vi "test hidde panel.vi"(8 "error in (no error)":errorcluster, 11 "TestCase in":refnum<class "Test Osciloscope Module.lvclass">) -> (0 "error out":errorcluster, 3 "TestCase out":refnum<class "Test Osciloscope Module.lvclass">)   [LabVIEW 2020, in "Test Osciloscope Module.lvclass"]
uses:
  Test Osciloscope Module.lvclass
  Test Osciloscope Module.lvclass/Test Osciloscope Module.ctl
  <vilib>/addons/_JKI Toolkits/VI Tester/TestCase.llb/TestCase.lvclass
  Libraries/Osciloscope/Osciloscope.lvlib
  C:/Program Files (x86)/National Instruments/LabVIEW 2020/vi.lib/addons/_JKI Toolkits/VI Tester/TestCase.llb/TestCase.lvclass
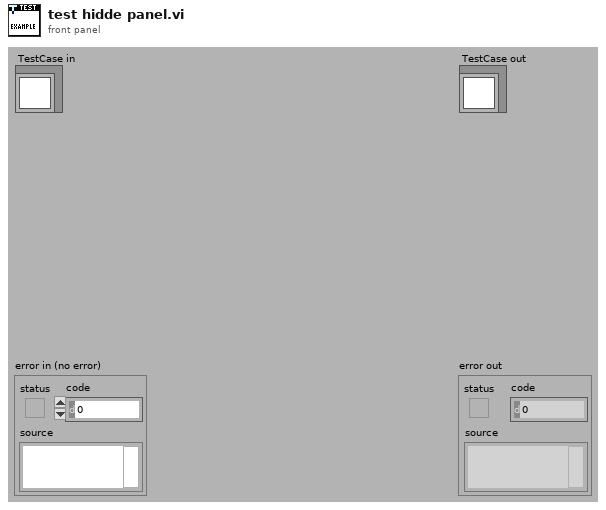
[diagram p1: front panel]
types:
  T1 = typedef "Osciloscope.lvlib/Broadcast Events--cluster.ctl" = cluster{"Module Did Init":refnum<user-event>, "Status Updated":refnum<user-event>, "Error Reported":refnum<user-event>, "Module Did Stop":refnum<user-event>, "Update Module Execution Status":refnum<user-event>, "Obtain Osciloscope Name":refnum<user-event>}
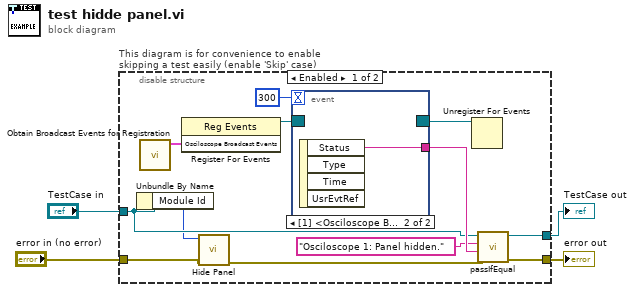
[diagram p0: block diagram]
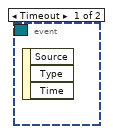
[diagram p2: hidden frame]
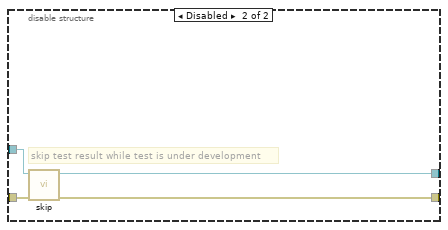
[diagram p3: hidden frame]
diagram:
  n1 = disable-structure "This diagram is for convenience to enable skipping a test easily (enable 'Skip' case)" shown="Enabled" {
    disable-tunnel: "TestCase in" -> [w6 w21]
    disable-tunnel: [w16 w19] -> w1
    disable-tunnel: [w15 w20] -> w3
    disable-tunnel: "error in (no error)" -> [w8 w18]
    frame Enabled {
      n2 = Unbundle By Name(w6) -> ("Module Id"=w5:i32)
      n3 = call "Obtain Broadcast Events for Registration.vi"() -> ("Osciloscope Broadcast Events"=w11:T1)  [unwired: 9 in, 2 out]
      n4 = register-events(w11) -> (reference out=w13:refnum<event-registration>)  [unwired: 2 in, 1 out]
      n5 = call "Hide Panel.vi"("error in (no error)"=w8, "Module ID"=w5) -> ("error out"=w7:errorcluster)  [unwired: 9 in]
      n6 = event shown="[1] <Osciloscope Broadcast Events.Status Updated>: User Event" {
        selector: w13 -> [_ _]
        dyn-events: [_ _] -> w14
        timeout: 300 -> [_ _]
        tunnel: [_ w17] -> w10
        event Timeout {
          n7 = event-data() -> ()  [unwired: 1 in, 3 out]
        }
        event User Event {
          n8 = event-data() -> ("Status"=w17:string)  [unwired: 1 in, 3 out]
        }
      }
      n9 = Unregister For Events(event registration refnum=w14) -> ()  [unwired: 1 in, 1 out]
      n10 = call-dynamic "passIfEqual.vi"("error in (no error)"=w7, "y"=w10, "x"="Osciloscope 1: Panel hidden.", "TestCase in"=w6) -> ("error out"=w15:errorcluster, "TestCase out"=w16:refnum<class "Test Osciloscope Module.lvclass">)  [unwired: 6 in]
    }
    frame Disabled {
      # "skip test result while test is under development"
      n11 = call <vilib>:"skip.vi"("error in (no error)"=w18, "TestCase in"=w21) -> ("error out"=w20:errorcluster, "TestCase out"=w19:refnum<class "Test Osciloscope Module.lvclass">)  [unwired: 8 in]
    }
  }
  "error out" <- w3
  "TestCase out" <- w1
